vi "CreateReplace Attribute.vi"(5 "Replace Existing (F)":bool, 6 "HDF5 Property List Ref":T1, 7 "Name":string, 8 "error in (no error)":errorcluster, 9 "HDF5 Dataspace Ref":T1, 10 "HDF5 Datatype Ref":T1, 11 "HDF5 Ref":T1) -> (0 "error out":errorcluster, 2 "HDF5 Attr Ref":T1, 3 "HDF5 Ref out":T1)   [LabVIEW 2017]
doc: "Creates or replaces an attribute on an HDF5 object"
uses:
  <vilib>/UPVI/lvhdf5/library.llb/HDF5 Ref.ctl
panel:
  # "LVHDF5 Toolkit\nCopyright (c) 2005-2013 by Jason D. Sommerville\nCopyright (c) 2014 by UPVI, LLC.\n\nThis use and distribution of this file is governed by the terms found in \nLICENSE.txt distributed with this toolkit and installed at\n <user.lib>\\_lvhdf5\\LICENSE.txt"
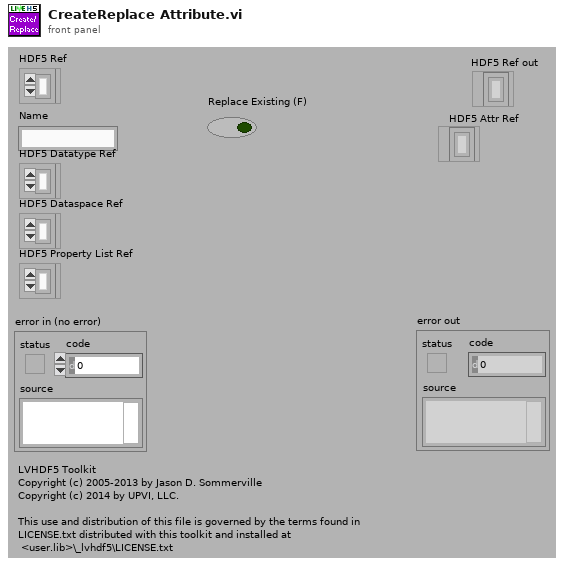
[diagram p1: front panel]
types:
  T1 = typedef "HDF5 Ref.ctl" = refnum<k1>
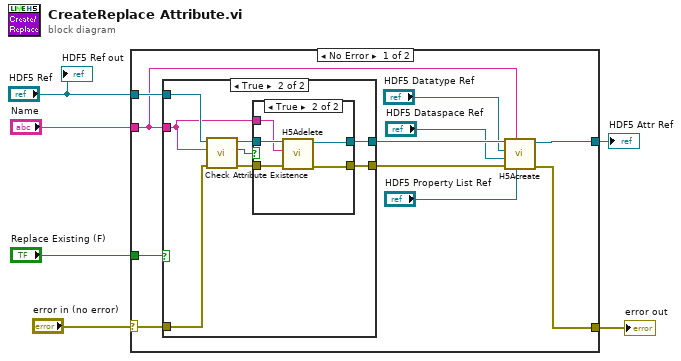
[diagram p0: block diagram]
diagram:
  n1 = case shown="No Error" "error in (no error)" {
    selector: "error in (no error)" -> [w15 w35]
    tunnel: [w7 w35] -> w5
    tunnel: "HDF5 Ref" -> [w16 _]
    tunnel: "Replace Existing (F)" -> [w17 _]
    tunnel: "Name" -> [w12 _]
    tunnel: [w8 _] -> w1
    frame No Error {
      n2 = case shown="True" w17 {
        tunnel: w16 -> [w19 w27]
        tunnel: w12 -> [_ w23]
        tunnel: w15 -> [w18 w26]
        tunnel: [w19 w21] -> w13
        tunnel: [w18 w20] -> w14
        frame False {
        }
        frame True {
          n3 = call <vilib>:"Check Attribute Existence.vi"("error in (no error)"=w26, "name"=w23, "HDF5 Ref"=w27) -> ("error out"=w24:errorcluster, "Exists"=w22:bool, "HDF5 Ref out"=w25:T1)  [unwired: 4 in]
          n4 = case shown="True" w22 {
            tunnel: w25 -> [w29 w34]
            tunnel: w24 -> [w28 w33]
            tunnel: w23 -> [_ w32]
            tunnel: [w29 w31] -> w21
            tunnel: [w28 w30] -> w20
            frame False {
            }
            frame True {
              n5 = call <vilib>:"H5Adelete.vi"("error in (no error)"=w33, "name"=w32, "HDF5 Ref"=w34) -> ("error out"=w30:errorcluster, "HDF5 Ref out"=w31:T1)  [unwired: 5 in]
            }
          }
        }
      }
      n6 = call <vilib>:"H5Acreate.vi"("HDF5 Create Property List Ref"="HDF5 Property List Ref", "Name"=w12, "error in (no error)"=w14, "HDF5 Dataspace Ref"="HDF5 Dataspace Ref", "HDF5 Datatype Ref"="HDF5 Datatype Ref", "HDF5 Location Ref"=w13) -> ("error out"=w7:errorcluster, "HDF5 Attr Ref"=w8:T1)  [unwired: 4 in]
    }
    frame Error {
    }
  }
  "error out" <- w5
  "HDF5 Attr Ref" <- w1
  "HDF5 Ref out" <- "HDF5 Ref"
